vi "ErrorMessages.vi"(8 "Fehler (Eingang, kein Fehler)":errorcluster, 11 "Errors":T2) -> (0 "error out":errorcluster, 3 "Error Array":T1(array[cluster]))   [LabVIEW 2020, in "Linearisierung v2.lvlib" / "SpanEinstellungen.lvlib"]
uses:
  SpanEinstellungen.lvlib
  LIN ErrorCluster.ctl
  Linearisierung v2.lvlib
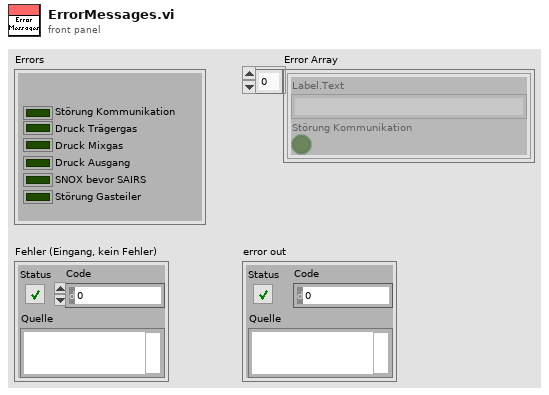
[diagram p1: front panel]
types:
  T1 = cluster{"Label.Text":string, "Störung Kommunikation":bool}[]
  T2 = typedef "Linearisierung v2.lvlib/LIN ErrorCluster.ctl" = cluster{"Störung Kommunikation":bool, "Pressure carrier gas":bool, "Pressure diluted gas":bool, "Outlet Pressure":bool, "SNOX before SAIR":bool, "Störung Gasteiler":bool}
  T3 = cluster{"Label.Text":string, "Störung Kommunikation":bool}
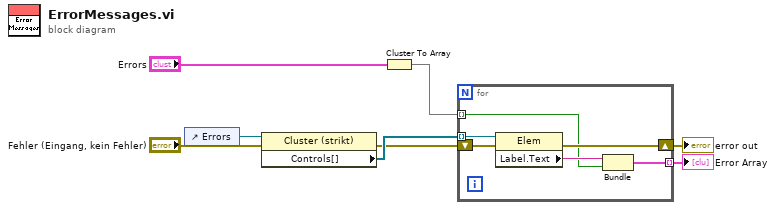
[diagram p0: block diagram]
diagram:
  n1 = control-ref of="Errors"() -> (w8:refnum<vi>)
  n2 = property class="Cluster (strikt)"(reference=w8, error in="Fehler (Eingang, kein Fehler)") -> (error out=w4:errorcluster, "Controls[]"=w7:refnum<vi>[])  [unwired: 1 out]
  n3 = Cluster To Array(cluster="Errors") -> (array=w2:bool[])
  n4 = for {
    tunnel: w7 -> [w14] mode=indexing
    shift-right: [w12] -> w3
    shift-left: w4 -> [w13]
    tunnel: w2 -> [w9] mode=indexing
    tunnel: [w10] -> w1 mode=indexing
    n5 = property class="Elem"(reference=w14, error in=w13) -> (error out=w12:errorcluster, "Label.Text"=w11:string)  [unwired: 1 out]
    n6 = Bundle("Label.Text"=w11, "Störung Kommunikation"=w9) -> (w10:T3)  [unwired: 1 in]
  }
  "error out" <- w3
  "Error Array" <- w1
